vi "Deney 5.vi"() -> ()   [LabVIEW 2018]
uses:
  <vilib>/measure/madcrms.llb/Basic Averaged DC-RMS for 1 Chan.vi
  <vilib>/measure/NI_MAPro.lvlib
panel:
  out "average":dbl format="%0.2p"
  out "rms value":dbl format="%0.2f"
  out "min value":dbl
  out "max value":dbl
  in  "stop":bool
  out "örnek sayısı":i32
  out "Path":path
  out "Waveform Graph":cluster{dbl, dbl, dbl[]}(graph)
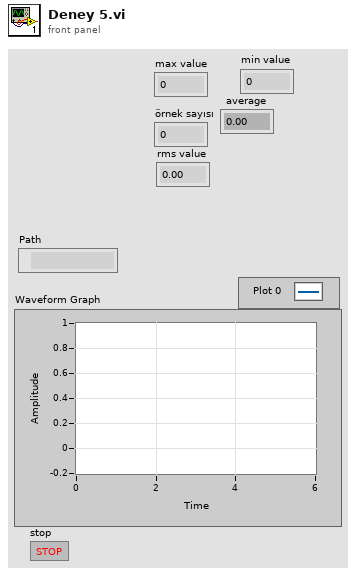
[diagram p1: front panel]
types:
  T1 = enum16{"open", "replace", "create", "open or create", "replace or create", "replace or create with confirmation"}
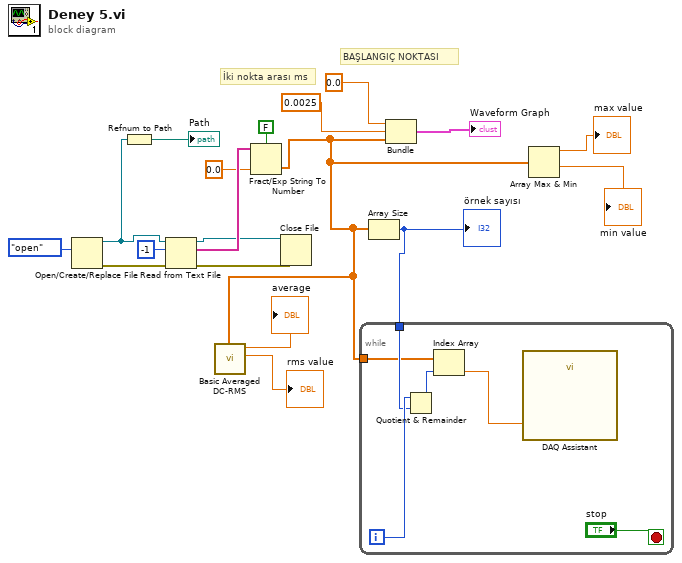
[diagram p0: block diagram]
diagram:
  # "İki nokta arası ms"
  # "BAŞLANGIÇ NOKTASI"
  n1 = Open/Create/Replace File(operation (0:open)=T1."open") -> (refnum out=w16:refnum<file>, error out=w18:errorcluster)  [unwired: 5 in, 1 out]
  n2 = Refnum to Path(1:w16) -> (0:→"Path":path)
  n3 = Read from Text File(file (use dialog)=w16, count=-1, error in=w18) -> (refnum out=w12:refnum<file>, text=w14:string[], error out=w11:errorcluster)  [unwired: 1 in, 1 out]
  n4 = Fract/Exp String To Number(use system decimal point (T)=FALSE, string=w14, default (0 dbl)=0.0 ("default (0 DBL)")) -> (number=w2:dbl[])  [unwired: 1 in, 1 out]
  n5 = call-poly <vilib>:"Basic Averaged DC-RMS.vi"("signal in"=w2) -> ("RMS value"=→"rms value":dbl, "DC value"=→"average":dbl)  [unwired: 7 in, 2 out]
  n6 = Close File(refnum=w12, error in=w11) -> ()  [unwired: 2 out]
  n7 = Array Size(array=w2) -> (size(s)=w8:i32)
  "örnek sayısı" <- w8
  n8 = while {
    tunnel: w2 -> [w21]
    tunnel: w8 -> [w23]
    i -> [w24]
    stop <- "stop" stop-if-true
    n9 = Quotient & Remainder(x=w24, y=w23) -> (x-y*floor(x/y)=w25:i32)  [unwired: 1 out]
    n10 = Index Array(array=w21, index=w25) -> (element=w20:dbl)
    n11 = call "DAQ Assistant"("data"=w20) -> ()  [unwired: 17 in, 2 out]
  }
  n12 = Bundle(0.0, 0.0025, w2) -> (→"Waveform Graph":cluster{dbl, dbl, dbl[]})  [unwired: 1 in]
  n13 = Array Max & Min(array=w2) -> (max value=→"max value":dbl, min value=→"min value":dbl)  [unwired: 2 out]
